vi "Get Output Assignements and Declarations.vi"(11 "output cluster":T1) -> (1 "output assignements, for multiframes":string[](array[string]), 2 "output declarations":string, 3 "outuput assignements":string)   [LabVIEW 2018]
doc: "Get output C code assignements and declarations for variables, to be able pass data to structures as ForLoop, WhileLoop, CaseStructure."
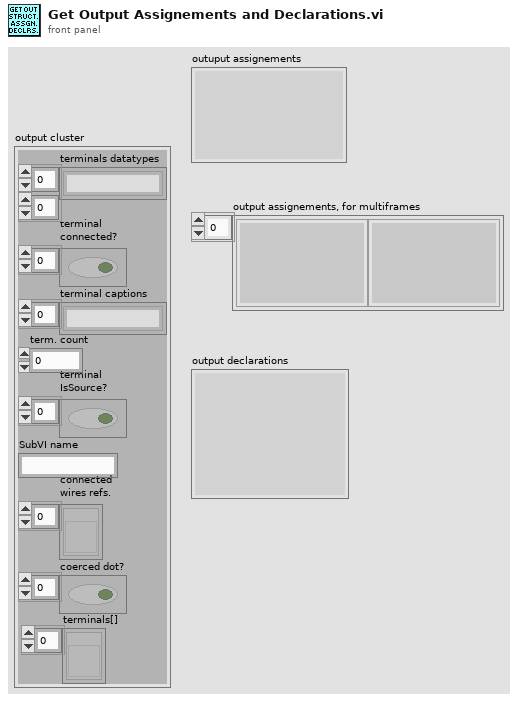
[diagram p1: front panel]
types:
  T1 = cluster{"terminals datatypes":string[][], "terminal\nconnected?":bool[], "terminal captions":string[], "term. count":i32, "terminal\nIsSource?":bool[], "SubVI name":string, "connected\nwires refs.":refnum<vi>[], "coerced dot?":bool[], "terminals[]":refnum<vi>[]}
  T2 = cluster{"wire labels":string[], "wire terminals datatypes":string[][]}
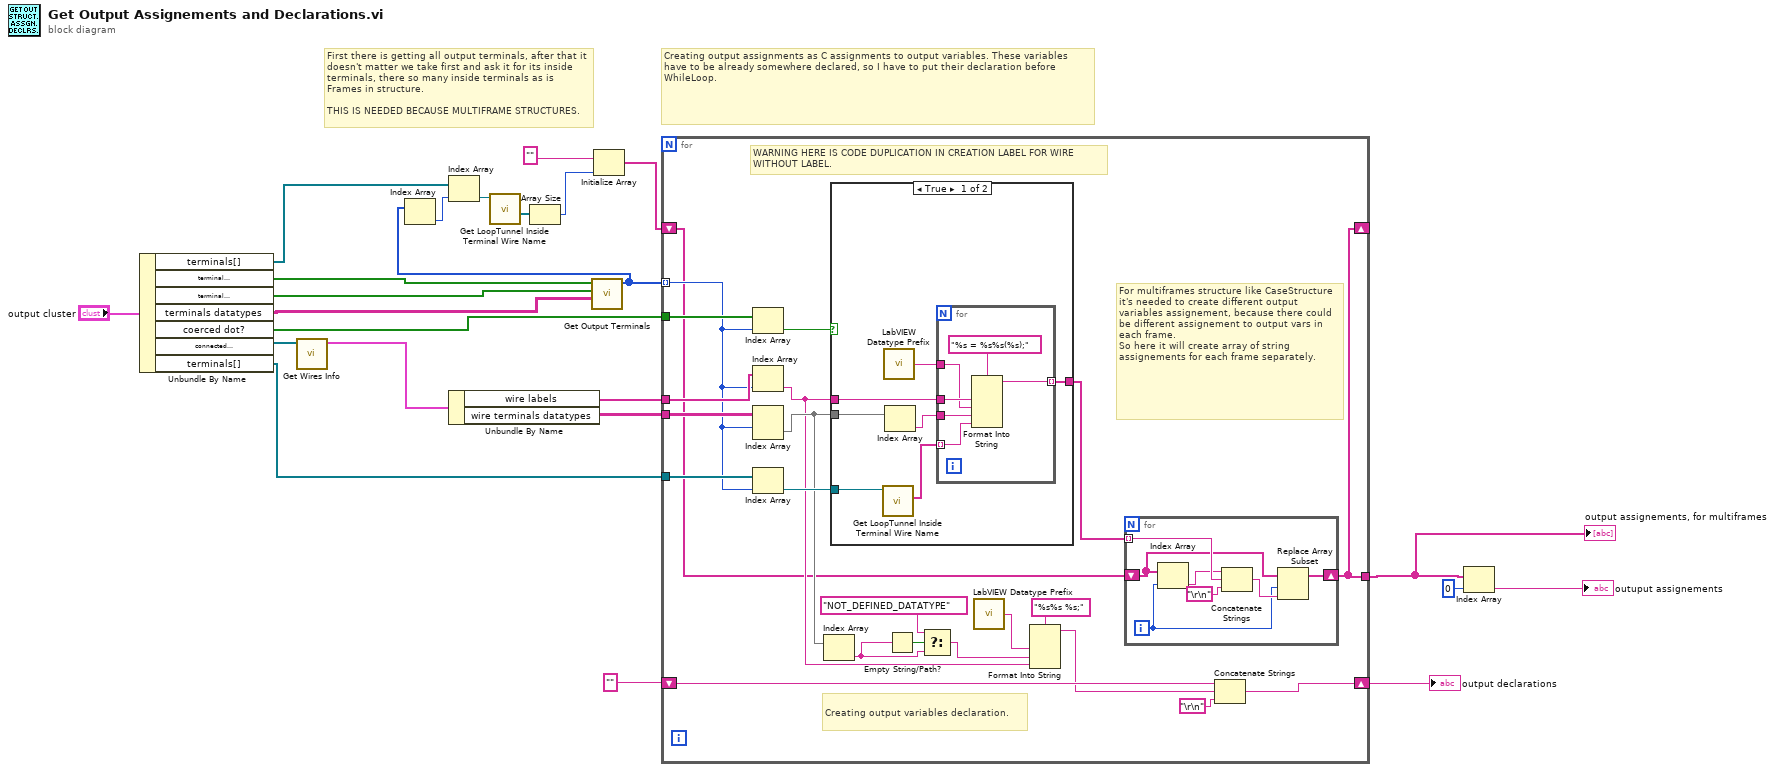
[diagram p0: block diagram]
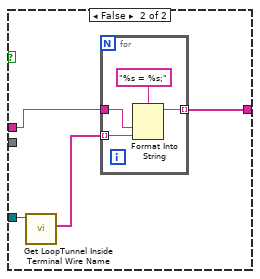
[diagram p2: hidden frame]
diagram:
  # "First there is getting all output terminals, after that it doesn't matter we take first and ask it for its inside terminals, there so many inside terminals as is Frames in structure.\n\nTHIS IS NEEDED BECAUSE MULTIFRAME STRUCTURES."
  # "Creating output assignments as C assignments to output variables. These variables have to be already somewhere declared, so I have to put their declaration before WhileLoop."
  n1 = Unbundle By Name("output cluster") -> ("terminals[]"=w3:refnum<vi>[], "terminal\nconnected?"=w22:bool[], "terminal\nIsSource?"=w23:bool[], "terminals datatypes"=w15:string[][], "coerced dot?"=w19:bool[], "connected\nwires refs."=w18:refnum<vi>[], "terminals[]"=w4:refnum<vi>[])
  n2 = call "Get Wires Info.vi"("connected\nwires refs."=w18) -> ("wires info cluster"=w17:T2)  [unwired: 10 in]
  n3 = Unbundle By Name(w17) -> ("wire labels"=w20:string[], "wire terminals datatypes"=w21:string[][])
  n4 = call "Get Output Terminals.vi"("terminals datatypes"=w15, "isSource?"=w23, "isConnected?"=w22) -> ("output terminals indexes"=w6:i32[])  [unwired: 8 in]
  n5 = Index Array(array=w6) -> (element=w5:i32)  [unwired: 1 in]
  n6 = Index Array(array=w3, index=w5) -> (element=w8:refnum<vi>)
  n7 = call "Get LoopTunnel Inside Terminal Wire Name.vi"("Terminal in"=w8) -> ("InsideTerms[]"=w2:refnum<vi>[])  [unwired: 8 in, 2 out]
  n8 = Array Size(array=w2) -> (size(s)=w1:i32)
  n9 = Initialize Array("", w1) -> (w7:string[])
  n10 = for {
    tunnel: w19 -> [w45]
    tunnel: w20 -> [w44]
    tunnel: w4 -> [w41]
    tunnel: w21 -> [w42]
    tunnel: w6 -> [w40] mode=indexing
    shift-right: [w29] -> w14
    shift-left: "" -> [w35]
    tunnel: [w26] -> w10
    shift-right: [w26] -> _
    shift-left: w7 -> [w27]
    # "For multiframes structure like CaseStructure it's needed to create different output variables assignement, because there could be different assignement to output vars in each frame.\nSo here it will create array of string assignements for each frame separately."
    # "Creating output variables declaration."
    # "WARNING HERE IS CODE DUPLICATION IN CREATION LABEL FOR WIRE WITHOUT LABEL."
    n11 = Index Array(array=w45, index=w40) -> (element=w43:bool)
    n12 = Index Array(array=w44, index=w40) -> (element=w36:string)
    n13 = Index Array(array=w42, index (row)=w40) -> (element=w37:string[])  [unwired: 1 in]
    n14 = Index Array(array=w41, index=w40) -> (element=w39:refnum<vi>)
    n15 = Index Array(array=w37) -> (element=w32:string)  [unwired: 1 in]
    n16 = case shown="True" w43 {
      tunnel: w36 -> [w59 w69]
      tunnel: w37 -> [w58 _]
      tunnel: w39 -> [w56 w68]
      tunnel: [w54 w66] -> w28
      frame True {
        n17 = call "Get LoopTunnel Inside Terminal Wire Name.vi"("Terminal in"=w56) -> ("LoopTunnel inside wire names"=w55:string[])  [unwired: 8 in, 2 out]
        n18 = call "LabVIEW Datatype Prefix.vi"() -> ("datatype prefix"=w53:string)
        n19 = Index Array(array=w58) -> (element=w57:string)  [unwired: 1 in]
        n20 = for {
          tunnel: w59 -> [w64]
          tunnel: w57 -> [w63]
          tunnel: w55 -> [w62] mode=indexing
          tunnel: [w61] -> w54 mode=indexing
          tunnel: w53 -> [w60]
          n21 = Format Into String(format string="%s = %s%s(%s);", w64, w60, w63, w62) -> (resulting string=w61:string)  [unwired: 2 in, 1 out]
        }
      }
      frame False {
        n22 = call "Get LoopTunnel Inside Terminal Wire Name.vi"("Terminal in"=w68) -> ("LoopTunnel inside wire names"=w67:string[])  [unwired: 8 in, 2 out]
        n23 = for {
          tunnel: w67 -> [w70] mode=indexing
          tunnel: w69 -> [w72]
          tunnel: [w71] -> w66 mode=indexing
          n24 = Format Into String(format string="%s = %s;", w72, w70) -> (resulting string=w71:string)  [unwired: 2 in, 1 out]
        }
      }
    }
    n25 = Empty String/Path?(string/path=w32) -> (empty?=w33:bool)
    n26 = Select(t="NOT_DEFINED_DATATYPE", s=w33, f=w32) -> (s? t:f=w30:string)
    n27 = call "LabVIEW Datatype Prefix.vi"() -> ("datatype prefix"=w24:string)
    n28 = Format Into String(format string="%s%s %s;", w24, w30, w36) -> (resulting string=w34:string)  [unwired: 2 in, 1 out]
    n29 = for {
      tunnel: w28 -> [w52] mode=indexing
      shift-right: [w49] -> w26
      shift-left: w27 -> [w47]
      i -> [w48]
      n30 = Index Array(array=w47, index=w48) -> (element=w51:string)
      n31 = Concatenate Strings(w51, w52, "\r\n") -> (w50:string)
      n32 = Replace Array Subset(array=w47, new element=w50, index=w48) -> (w49:string[])
    }
    n33 = Concatenate Strings(w35, w34, "\r\n") -> (w29:string)
  }
  "output declarations" <- w14
  "output assignements, for multiframes" <- w10
  n34 = Index Array(array=w10, index=0 ("index (row)")) -> (element=→"outuput assignements":string)
